vi "Set CCMD DSP402.vi"(2 "error in (no error)":errorcluster, 3 "DSP402 in":refnum<class "DSP402.lvclass">) -> (0 "error out":errorcluster, 1 "DSP402 out":refnum<class "DSP402.lvclass">)   [LabVIEW 2017, in "canopen.lvlib" / "DSP402.lvclass"]
uses:
  DSP402.lvclass
  DSP402.lvclass/DSP402.ctl
  CANopen/Multiplexor.ctl
  Download DSP402 (U16).vi
  CANopen/CANopen.lvclass
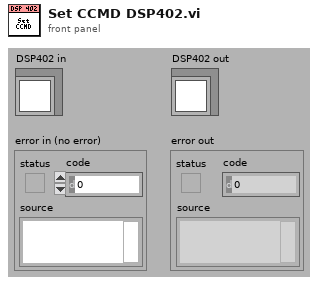
[diagram p1: front panel]
types:
  T1 = typedef "canopen.lvlib/CANopen.lvclass/Multiplexor.ctl" = cluster{"Index":u16, "Sub-index":u8}
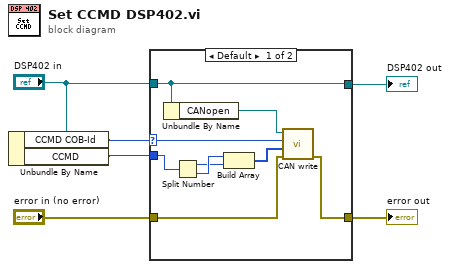
[diagram p0: block diagram]
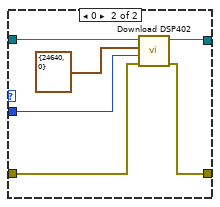
[diagram p2: hidden frame]
diagram:
  n1 = Unbundle By Name("DSP402 in") -> ("CCMD COB-Id"=w1:u32, "CCMD"=w2:u16)
  n2 = case shown="Default" w1 {
    selector: w1 -> [w12 _]
    tunnel: "error in (no error)" -> [w15 w21]
    tunnel: [w14 w19] -> w5
    tunnel: w2 -> [w10 w17]
    tunnel: "DSP402 in" -> [w13 w18]
    tunnel: [w13 w16] -> w3
    frame Default {
      n3 = Unbundle By Name(w13) -> ("CANopen"=w11:refnum<class "CANopen.lvclass">)
      n4 = Split Number(x=w10) -> (hi(x)=w8:u8, lo(x)=w9:u8)
      n5 = Build Array(w9, w8) -> (w7:u8[])
      n6 = call "CAN write.vi"("error in (no error)"=w15, "Data"=w7, "COB id"=w12, "CANopen in"=w11) -> ("error out"=w14:errorcluster)  [unwired: 3 out]
    }
    frame 0 {
      n7 = call-poly "Download DSP402.vi"("error in (no error)"=w21, "Value"=w17, "Multiplexor"=T1 {"Index"=24640, "Sub-index"=0}, "DSP402 in"=w18) -> ("error out"=w19:errorcluster, "DSP402 out"=w16:refnum<class "DSP402.lvclass">)  [unwired: 1 in, 1 out]
    }
  }
  "error out" <- w5
  "DSP402 out" <- w3
